vi "FL Implication COA.vi"(5 "user MF interpolating polynomials":T1[](array[typedef]) {"coa_x(y) coeff" format="%.4g"; "Area(y) coeff" format="%.4g"; "X(y) coeff" format="%.4g"; "Y(x) coeff" format="%.4g"; "Y" format="%.4g"; "X" format="%.4g"}, 6 "user-defined \nshape index":i32, 7 "Function":T2=10 items=["Triangle", "Trapezoid", "Singleton", "Sigmoid", "Gaussian", "User-Defined"], 9 "Weight":dbl, 10 "Implication":T3 items=["Minimum", "Product"], 11 "Points (X)":dbl[](array[numeric])) -> (0 "area":dbl, 3 "X(CoA)":dbl)   [LabVIEW 2017, in "NI_Fuzzy_Logic_API.lvlib"]
uses:
  <vilib>/addons/Fuzzy Logic/NI_Fuzzy_Logic_API.lvlib
  <vilib>/addons/Fuzzy Logic/TypeDefs/FL Consequent Implication.ctl
  <vilib>/addons/Fuzzy Logic/TypeDefs/FL Membership Function Shape.ctl
  <vilib>/addons/Fuzzy Logic/TypeDefs/FL Interpolating polynomials.ctl
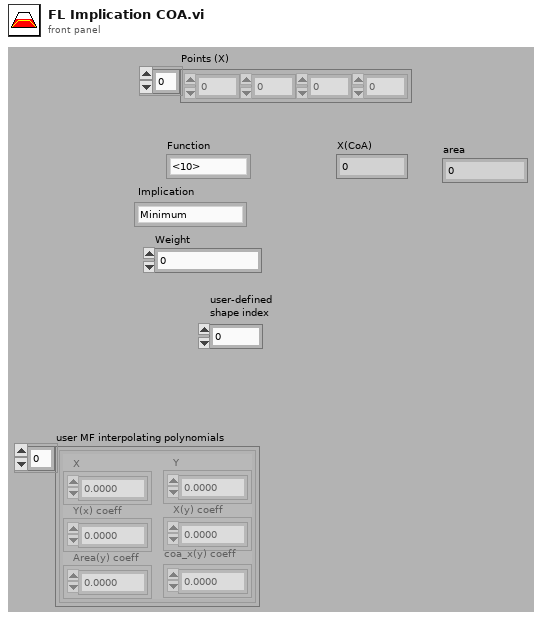
[diagram p1: front panel]
types:
  T1 = typedef "NI_Fuzzy_Logic_API.lvlib/FL Interpolating polynomials.ctl" = cluster{"X":dbl[], "Y":dbl[], "Y(x) coeff":dbl[][], "X(y) coeff":dbl[][], "Area(y) coeff":dbl[][], "coa_x(y) coeff":dbl[][]}
  T2 = typedef "NI_Fuzzy_Logic_API.lvlib/FL Membership Function Shape.ctl" = u16
  T3 = typedef "NI_Fuzzy_Logic_API.lvlib/FL Consequent Implication.ctl" = u16
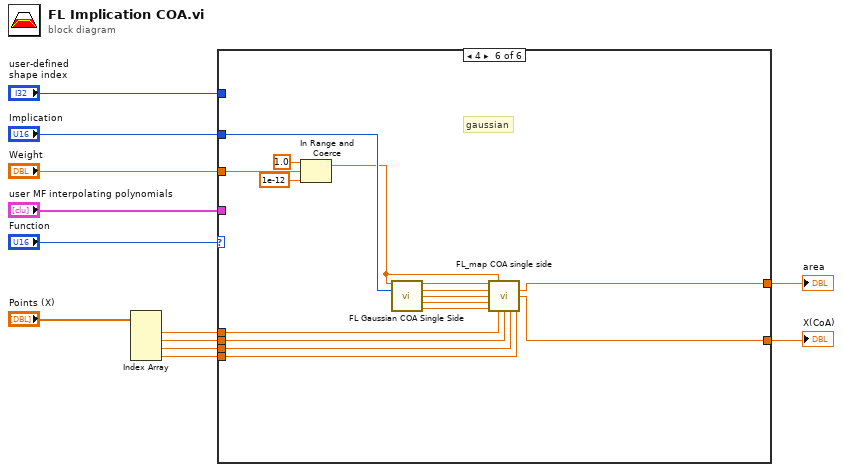
[diagram p0: block diagram]
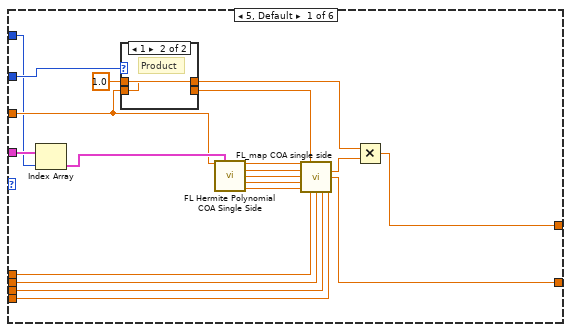
[diagram p2: hidden frame]
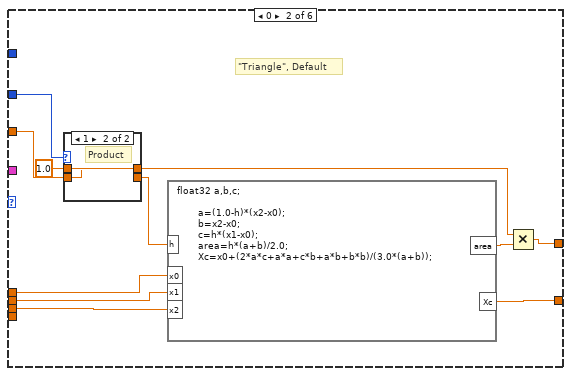
[diagram p4: hidden frame]
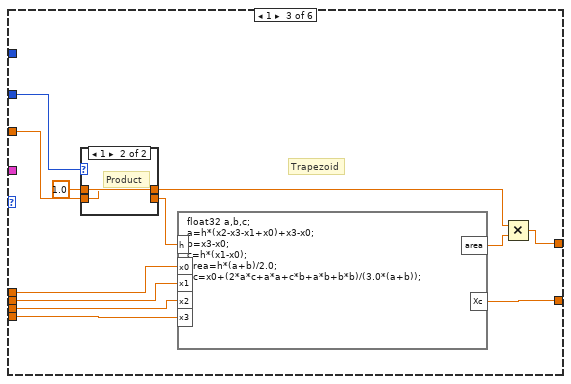
[diagram p6: hidden frame]
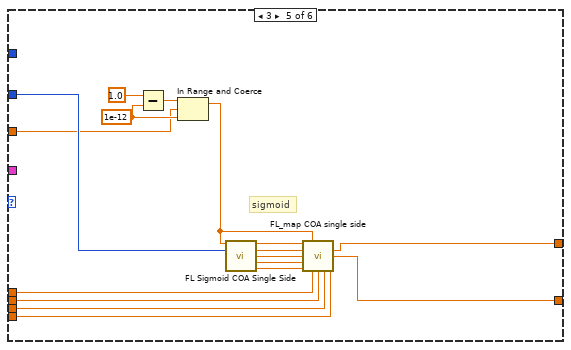
[diagram p9: hidden frame]
diagram:
  n1 = Index Array(array="Points (X)") -> (element #1=w6:dbl, element #2=w5:dbl, element #3=w4:dbl, element #4=w3:dbl)  [unwired: 4 in]
  n2 = case shown="4" "Function" {
    tunnel: "Weight" -> [w19 w42 w56 w68 w71 w88]
    tunnel: [w27 w47 w63 w69 w78 w93] -> w9
    tunnel: [w23 w37 w53 w68 w76 w94] -> w7
    tunnel: w6 -> [w31 w46 w62 w69 w82 w98]
    tunnel: w5 -> [w30 w45 w61 _ w81 w97]
    tunnel: w4 -> [w29 w44 w60 _ w80 w96]
    tunnel: w3 -> [w28 _ w59 _ w79 w95]
    tunnel: "user MF interpolating polynomials" -> [w32 _ _ _ _ _]
    tunnel: "Implication" -> [w26 w41 w57 _ w75 w92]
    tunnel: "user-defined \nshape index" -> [w13 _ _ _ _ _]
    frame 5, Default {
      n3 = Index Array(array=w32, index=w13) -> (element=w20:T1)
      n4 = case shown="1" w26 {
        tunnel: w19 -> [w33 w35]
        tunnel: 1.0 -> [w34 w36]
        tunnel: [w34 w35] -> w22
        tunnel: [w33 w36] -> w21
        frame 0, Default {
          # "Min"
        }
        frame 1 {
          # "Product"
        }
      }
      n5 = call <vilib>:"FL Hermite Polynomial COA Single Side.vi"("weight"=w19, "element"=w20) -> ("xlh"=w18:dbl, "area"=w17:dbl, "coa_x"=w16:dbl, "x_l"=w15:dbl, "x_r"=w14:dbl)  [unwired: 1 in, 8 out]
      n6 = call <vilib>:"FL_map COA single side.vi"("xlh"=w18, "weight"=w21, "area"=w17, "coa_x"=w16, "x_l"=w15, "x_r"=w14, "x0"=w31, "x1"=w30, "x2"=w29, "x3"=w28) -> ("area"=w24:dbl, "coa_x"=w27:dbl)  [unwired: 4 out]
      n7 = Multiply(x=w22, y=w24) -> (x*y=w23:dbl)
    }
    frame 0 {
      # "\"Triangle\", Default"
      n8 = case shown="1" w41 {
        tunnel: w42 -> [w48 w50]
        tunnel: 1.0 -> [w49 w51]
        tunnel: [w49 w50] -> w39
        tunnel: [w48 w51] -> w40
        frame 0, Default {
          # "Min"
        }
        frame 1 {
          # "Product"
        }
      }
      n9 = formula code="float32 a,b,c;\n\n       a=(1.0-h)*(x2-x0);\n       b=x2-x0;\n       c=h*(x1-x0);\n       area=h*(a+b)/2.0;\n       Xc=x0+(2*a*c+a*a+c*b+a*b+b*b)/(3.0*(a+b));"("x0"=w46, "x1"=w45, "x2"=w44, "h"=w40) -> ("area"=w38:dbl, "Xc"=w47:dbl)
      n10 = Multiply(x=w39, y=w38) -> (x*y=w37:dbl)
    }
    frame 1 {
      # "Trapezoid"
      n11 = case shown="1" w57 {
        tunnel: w56 -> [w64 w66]
        tunnel: 1.0 -> [w65 w67]
        tunnel: [w65 w66] -> w52
        tunnel: [w64 w67] -> w55
        frame 0, Default {
          # "Min"
        }
        frame 1 {
          # "Product"
        }
      }
      n12 = formula code="float32 a,b,c;\na=h*(x2-x3-x1+x0)+x3-x0;\nb=x3-x0;\nc=h*(x1-x0);\narea=h*(a+b)/2.0;\nXc=x0+(2*a*c+a*a+c*b+a*b+b*b)/(3.0*(a+b));"("x0"=w62, "x1"=w61, "x2"=w60, "h"=w55, "x3"=w59) -> ("area"=w54:dbl, "Xc"=w63:dbl)
      n13 = Multiply(x=w52, y=w54) -> (x*y=w53:dbl)
    }
    frame 2 {
      # "singleton"
    }
    frame 3 {
      w73 = 1e-12 ("lower limit")
      # "sigmoid"
      n14 = Subtract(x=1.0, y=w73) -> (x-y=w72:dbl)
      n15 = In Range and Coerce(upper limit=w72, x=w71, lower limit=w73) -> (coerced(x)=w70:dbl)  [unwired: 1 out]
      n16 = call <vilib>:"FL Sigmoid COA Single Side.vi"("weight"=w70, "Implication"=w75) -> ("xlh"=w77:dbl, "area"=w86:dbl, "coa_x"=w85:dbl, "x_l"=w84:dbl, "x_r"=w83:dbl)  [unwired: 3 in, 6 out]
      n17 = call <vilib>:"FL_map COA single side.vi"("xlh"=w77, "weight"=w70, "area"=w86, "coa_x"=w85, "x_l"=w84, "x_r"=w83, "x0"=w82, "x1"=w81, "x2"=w80, "x3"=w79) -> ("area"=w76:dbl, "coa_x"=w78:dbl)  [unwired: 4 out]
    }
    frame 4 {
      # "gaussian"
      n18 = In Range and Coerce(upper limit=1.0, x=w88, lower limit=1e-12) -> (coerced(x)=w87:dbl)  [unwired: 1 out]
      n19 = call <vilib>:"FL Gaussian COA Single Side.vi"("weight"=w87, "Implication"=w92) -> ("xlh"=w91:dbl, "area"=w102:dbl, "coa_x"=w101:dbl, "x_l"=w100:dbl, "x_r"=w99:dbl)  [unwired: 9 out]
      n20 = call <vilib>:"FL_map COA single side.vi"("xlh"=w91, "weight"=w87, "area"=w102, "coa_x"=w101, "x_l"=w100, "x_r"=w99, "x0"=w98, "x1"=w97, "x2"=w96, "x3"=w95) -> ("area"=w94:dbl, "coa_x"=w93:dbl)  [unwired: 4 out]
    }
  }
  "X(CoA)" <- w9
  "area" <- w7
